vi "Main.vi"() -> ()   [LabVIEW 2015]
uses:
  <vilib>/Analysis/baseanly.llb/Mean (DBL).vi
  <vilib>/Analysis/NI_AALBase.lvlib
panel:
  out "x+y":dbl
  out "x/y":dbl
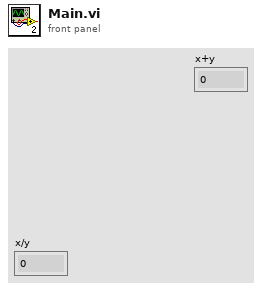
[diagram p1: front panel]
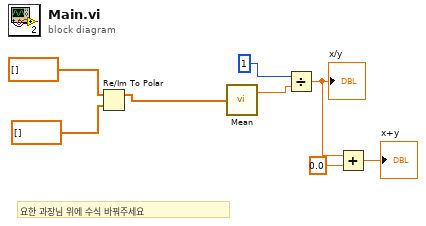
[diagram p0: block diagram]
diagram:
  # "요한 과장님 위에 수식 바꿔주세요"
  n1 = Re/Im To Polar(2:dbl[] [], 3:dbl[] []) -> (1:w6:dbl[])  [unwired: 1 out]
  n2 = call-poly <vilib>:"Mean.vi"("X"=w6) -> ("mean"=w5:dbl)  [unwired: 1 out]
  n3 = Divide(x=1, y=w5) -> (x/y=w3:dbl)
  "x/y" <- w3
  n4 = Add(x=w3, y=0.0) -> (x+y=→"x+y":dbl)
